vi "CODMn启动命令 (子VI).vi"(10 "CODMn量程切换":enum32{"H", "L", "AUTO"}(ring)=enum."AUTO", 11 "启动测量模式":T1) -> ()   [LabVIEW 2016, in "斯坦道CODMn.lvlib"]
uses:
  <vilib>/Plasmionique/MB Master/MB_Master_Serial/MB_Master_Serial.lvclass
  C:/Program Files (x86)/National Instruments/LabVIEW 2016/vi.lib/Plasmionique/MB Master/MB_Master/MB_Master.lvclass
  <vilib>/Plasmionique/MB Master/MB Master.lvlib
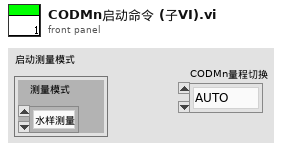
[diagram p1: front panel]
types:
  T1 = cluster{"测量模式":enum16{"水样测量", "标样核查", "零点核查", "跨度核查", "空白测试", "加标回收", "平行样", "校零", "校标"}}
  T2 = cluster{"baud rate (bps)":u32, "stop bits":u16, "parity":u16, "flow control":u16, "timeout":u32, "retries":i32}
  T3 = enum16{"水样测量", "标样核查", "零点核查", "跨度核查", "空白测试", "加标回收", "平行样", "校零", "校标"}
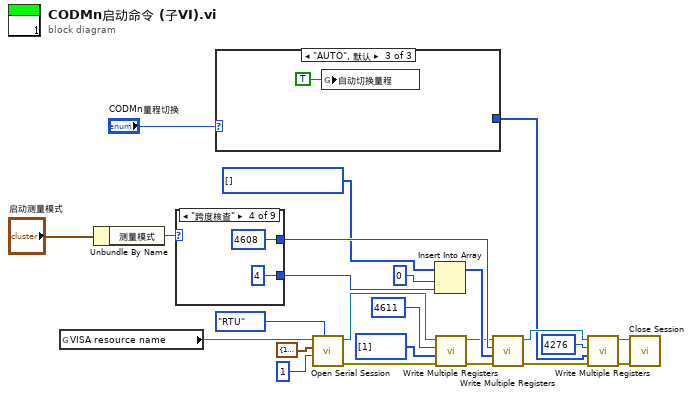
[diagram p0: block diagram]
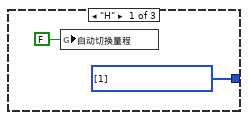
[diagram p2: hidden frame]
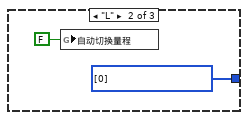
[diagram p3: hidden frame]
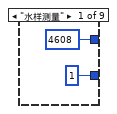
[diagram p4: hidden frame]
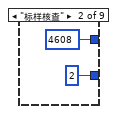
[diagram p5: hidden frame]
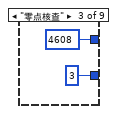
[diagram p6: hidden frame]
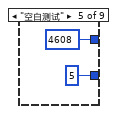
[diagram p7: hidden frame]
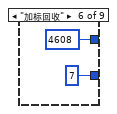
[diagram p8: hidden frame]
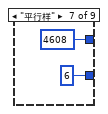
[diagram p9: hidden frame]
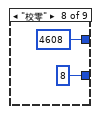
[diagram p10: hidden frame]
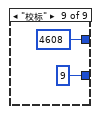
[diagram p11: hidden frame]
diagram:
  n1 = global read "COD浓度全局变量.vi" "VISA resource name"() -> (w7:refnum<visa-resource-name>)
  n2 = Unbundle By Name("启动测量模式") -> ("测量模式"=w19:T3)
  n3 = case shown="\"跨度核查\"" w19 {
    tunnel: [u16 4608 ("address") u16 4608 ("address") u16 4608 ("address") u16 4608 ("address") u16 4608 ("address") u16 4608 ("address") u16 4608 ("address") u16 4608 ("address") u16 4608 ("address")] -> w23
    tunnel: [u16 1 ("address") u16 2 ("address") u16 3 ("address") u16 4 ("address") u16 5 ("address") u16 7 ("address") u16 6 ("address") u16 8 ("address") u16 9 ("address")] -> w17
    frame "水样测量" {
    }
    frame "标样核查" {
    }
    frame "零点核查" {
    }
    frame "跨度核查" {
    }
    frame "空白测试" {
    }
    frame "加标回收" {
    }
    frame "平行样" {
    }
    frame "校零" {
    }
    frame "校标" {
    }
  }
  n4 = case shown="\"AUTO\", 默认" "CODMn量程切换" {
    tunnel: [u16[] [1] ("values") u16[] [0] ("values") _] -> w8
    frame "H" {
      n5 = global write "系统变量.vi" "自动切换量程"(FALSE ("自动切换量程")) -> ()
    }
    frame "L" {
      n6 = global write "系统变量.vi" "自动切换量程"(FALSE ("自动切换量程")) -> ()
    }
    frame "AUTO", Default {
      n7 = global write "系统变量.vi" "自动切换量程"(TRUE ("自动切换量程")) -> ()
    }
  }
  n8 = call <vilib>:"Open Serial Session.vi"("Mode (RTU)"=enum16{"RTU", "ASCII"}."RTU", "Slave ID"=u8 1, "Serial Config"=T2 {"baud rate (bps)"=115200, "stop bits"=10, "parity"=0, "flow control"=0, "timeout"=1000, "retries"=1}, "VISA Resource"=w7) -> ("Error out"=w4:errorcluster, "MB_Serial session"=w6:refnum<class "MB_Master_Serial.lvclass">)  [unwired: 6 in]
  n9 = Insert Into Array(array=u16[] [] ("values"), index=0 ("索引"), new element=w17) -> (w24:u16[])
  n10 = call <vilib>:"Write Multiple Registers.vi"("error in (no error)"=w4, "values"=u16[] [1], "starting address"=u16 4611, "MB session in"=w6) -> ("error out"=w3:errorcluster, "MB session out"=w5:refnum<class "MB_Master_Serial.lvclass">)  [unwired: 6 in]
  n11 = call <vilib>:"Write Multiple Registers.vi"("error in (no error)"=w3, "values"=w24, "starting address"=w23, "MB session in"=w5) -> ("error out"=w13:errorcluster, "MB session out"=w14:refnum<class "MB_Master_Serial.lvclass">)  [unwired: 6 in]
  n12 = call <vilib>:"Write Multiple Registers.vi"("error in (no error)"=w13, "values"=w8, "starting address"=u16 4276, "MB session in"=w14) -> ("error out"=w11:errorcluster, "MB session out"=w12:refnum<class "MB_Master_Serial.lvclass">)  [unwired: 6 in]
  n13 = call-dynamic "Close Session.vi"("error in (no error)"=w11, "MB_Serial session"=w12) -> ()  [unwired: 9 in, 1 out]
